vi "Is Created Event.vi"(10 "Created Event Alias":string, 11 "Template Queue in":refnum<class "Template Queue.lvclass">) -> (2 "Is Created Event?":bool, 3 "Template Queue out":refnum<class "Template Queue.lvclass">)   [LabVIEW 2021, in "Template Queue.lvlib" / "Template Queue.lvclass"]
uses:
  Template Queue.lvclass
  Template Queue.lvclass/Template Queue.ctl
  <vilib>/Nathan Davis/jettl/jettl/Queue/Queue.lvclass
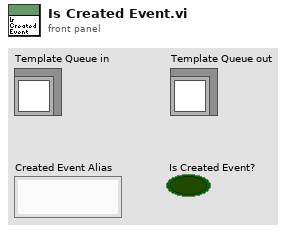
[diagram p1: front panel]
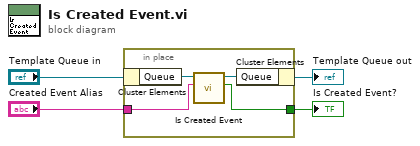
[diagram p0: block diagram]
diagram:
  n1 = in-place {
    in-place-border: [w6] -> w2
    in-place-border: "Created Event Alias" -> [w5]
    n2 = in-place-cluster #1("Template Queue in") -> ("Queue"=w8:refnum<class "Queue.lvclass">)
    n3 = call-dynamic "Is Created Event.vi"("Created Event Alias"=w5, "Queue in"=w8) -> ("Is Created Event?"=w6:bool, "Queue out"=w7:refnum<class "Queue.lvclass">)  [unwired: 8 in]
    n4 = in-place-cluster #1("Queue"=w7) -> (→"Template Queue out":refnum<class "Template Queue.lvclass">)
  }
  "Is Created Event?" <- w2
